vi "Read.vi"(11 "MultiError Value in":refnum<class "MultiError Value.lvclass">) -> (2 "MultiErrors":refnum<class "MultiErrors.lvclass">)   [LabVIEW 2020, in "Volatus.lvlib" / "MultiError Value.lvclass"]
uses:
  MultiError Value.lvclass
  MultiError Value.lvclass/MultiError Value.ctl
  MultiErrors/MultiErrors.lvclass
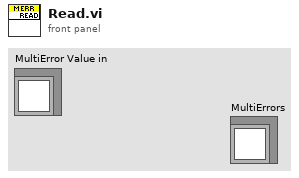
[diagram p1: front panel]
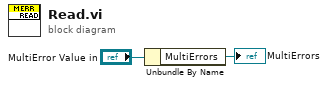
[diagram p0: block diagram]
diagram:
  n1 = Unbundle By Name("MultiError Value in") -> ("MultiErrors"=→"MultiErrors":refnum<class "MultiErrors.lvclass">)
